vi "WPS_inputCluster.vi"(0 "Input Cluster":T1) -> (1 "standard output":string, 2 "standard error":string, 3 "return code":i32, 4 "error out":errorcluster)   [LabVIEW 2016]
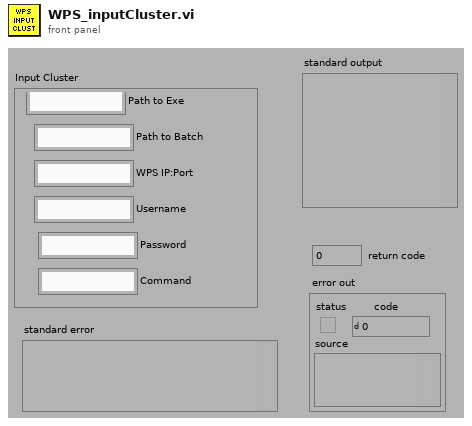
[diagram p1: front panel]
types:
  T1 = cluster{"Path to Batch":string, "WPS IP:Port":string, "Username":string, "Password":string, "Command":string, "Path to Exe":string}
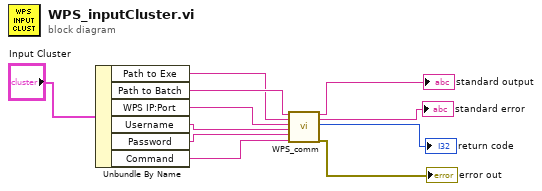
[diagram p0: block diagram]
diagram:
  n1 = Unbundle By Name("Input Cluster") -> ("Path to Exe"=w2:string, "Path to Batch"=w10:string, "WPS IP:Port"=w9:string, "Username"=w8:string, "Password"=w7:string, "Command"=w1:string)
  n2 = call "WPS_comm.vi"("Path to Batch"=w10, "Path to Exe"=w2, "WPS IP:Port"=w9, "Username"=w8, "Password"=w7, "Command"=w1) -> ("standard output"=→"standard output":string, "standard error"=→"standard error":string, "return code"=→"return code":i32, "error out"=→"error out":errorcluster)  [unwired: 10 in]
